vi "Noise_Tests.vi"(0 "tdms file in":refnum<k34>, 5 "Ch1_in":dbl[](array[numeric]), 7 "Ch2_in":dbl[](array[numeric]), 12 "group name":string, 13 "channel names":string[](array[string])) -> (4 "tdms file out":refnum<k34>, 6 "Ch1_out":dbl[](array[numeric]), 8 "Ch2_out":dbl[](array[numeric]), 10 "Hist":i32[][](array[numeric]), 14 "Noise Spectrum":T1(array[cluster]), 15 "Waveforms":waveform(dbl)[](array[waveform]))   [LabVIEW 2019]
uses:
  SiPM_Tests_Global_Var.vi
  <vilib>/Analysis/NI_AALPro.lvlib
  Agilent_lib/Agilent 2000 3000 X-Series.lvlib
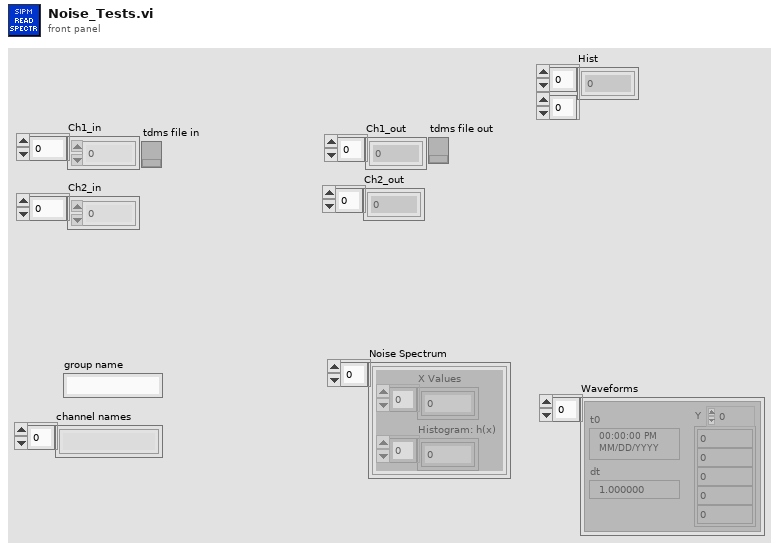
[diagram p1: front panel]
types:
  T1 = cluster{"X Values":dbl[], "Histogram: h(x)":i32[]}[]
  T2 = cluster{"X Values":dbl[], "Histogram: h(x)":i32[]}
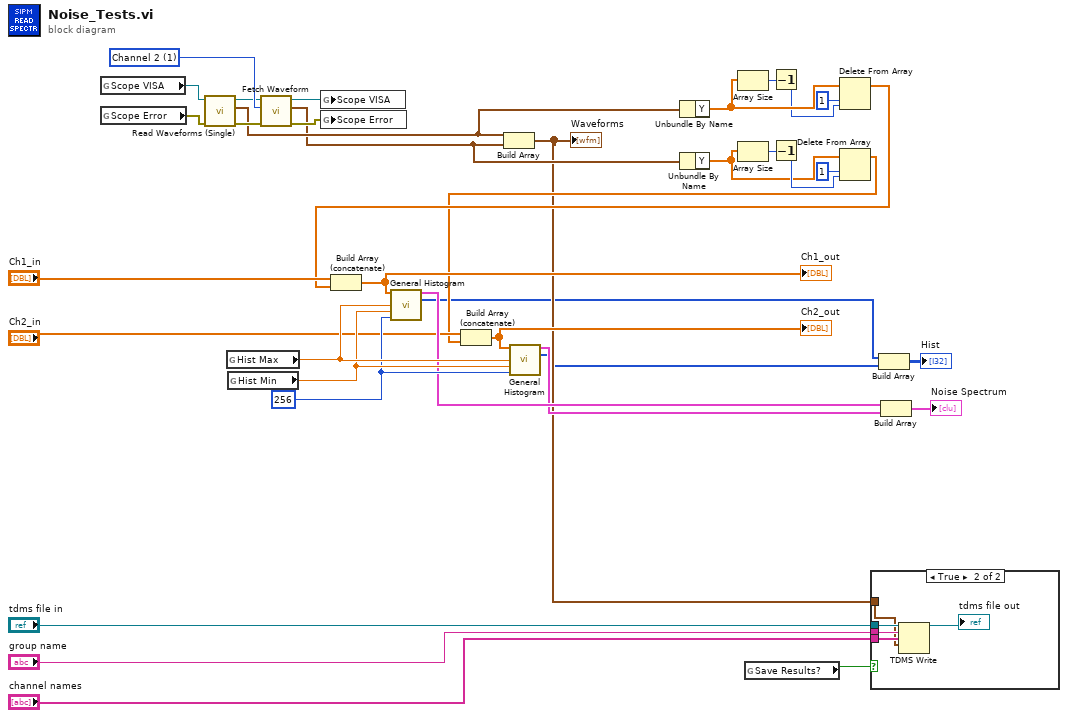
[diagram p0: block diagram]
diagram:
  w25 = 1 items=["Channel 1"=0, "Channel 2"=1, "Channel 3"=2, "Channel 4"=3, "Waveform Memory 1"=5, "Waveform Memory 2"=6, "Serial Bus 1"=7, "Serial Bus 2"=8, "Digital Bus Low"=9, "Digital Bus High "=10, "Digital Bus 1"=11, "Digital Bus 2"=12, "Function 1"=32, "Function 2"=33, "Function 3"=34, "Function 4"=35, "Math 1"=36, "Math 2"=37, "Math 3"=38, "Math 4"=39] ("Source Channel (0: Channel 1)")
  w32 = 256 ("# bins")
  n1 = global read "SiPM_Tests_Global_Var.vi" "Scope VISA"() -> (w21:refnum<visa-resource-name>)
  n2 = global read "SiPM_Tests_Global_Var.vi" "Scope Error"() -> (w22:errorcluster)
  n3 = call "Read Waveforms (Single).vi"("error in (no error)"=w22, "VISA resource name"=w21) -> ("error out"=w24:errorcluster, "Waveform Data"=w10:waveform(dbl), "VISA resource name out"=w23:refnum<visa-resource-name>)  [unwired: 7 in]
  n4 = global read "SiPM_Tests_Global_Var.vi" "Hist Max"() -> (w34:dbl)
  n5 = global read "SiPM_Tests_Global_Var.vi" "Hist Min"() -> (w33:dbl)
  n6 = call "Fetch Waveform.vi"("error in (no error)"=w24, "Source Channel (0: Channel 1)"=w25, "VISA resource name"=w23) -> ("error out"=w19:errorcluster, "Waveform Data"=w9:waveform(dbl), "VISA resource name out"=w20:refnum<visa-resource-name>)  [unwired: 2 in, 4 out]
  n7 = global write "SiPM_Tests_Global_Var.vi" "Scope VISA"(w20) -> ()
  n8 = global write "SiPM_Tests_Global_Var.vi" "Scope Error"(w19) -> ()
  n9 = Build Array(w10, w9) -> (w4:waveform(dbl)[])
  "Waveforms" <- w4
  n10 = Unbundle By Name(w10) -> ("Y"=w17:dbl[])
  n11 = Unbundle By Name(w9) -> ("Y"=w11:dbl[])
  n12 = Array Size(array=w17) -> (size(s)=w16:i32)
  n13 = Array Size(array=w11) -> (size(s)=w13:i32)
  n14 = global read "SiPM_Tests_Global_Var.vi" "Save Results?"() -> (w5:bool)
  n15 = Decrement(x=w16) -> (x-1=w15:i32)
  n16 = Decrement(x=w13) -> (x-1=w14:i32)
  n17 = Delete From Array(array=w17, length=1, index=w15) -> (array with subset deleted=w8:dbl[])  [unwired: 1 out]
  n18 = Build Array (concatenate)("Ch1_in", w8) -> (w36:dbl[])
  "Ch1_out" <- w36
  n19 = call <vilib>:"General Histogram.vi"("X"=w36, "max"=w34, "min"=w33, "# bins"=w32) -> ("Histogram Graph"=w31:T2, "Histogram"=w3:i32[])  [unwired: 7 in, 3 out]
  n20 = Delete From Array(array=w11, length=1, index=w14) -> (array with subset deleted=w6:dbl[])  [unwired: 1 out]
  n21 = Build Array (concatenate)("Ch2_in", w6) -> (w35:dbl[])
  "Ch2_out" <- w35
  n22 = call <vilib>:"General Histogram.vi"("X"=w35, "max"=w34, "min"=w33, "# bins"=w32) -> ("Histogram Graph"=w30:T2, "Histogram"=w2:i32[])  [unwired: 7 in, 3 out]
  n23 = case shown="True" w5 {
    tunnel: "tdms file in" -> [_ w41]
    tunnel: "group name" -> [_ w40]
    tunnel: "channel names" -> [_ w39]
    tunnel: w4 -> [_ w38]
    frame False {
    }
    frame True {
      n24 = TDMS Write(0:w41, 5:w40, 7:w39, 9:w38) -> (4:→"tdms file out":refnum<k34>)  [unwired: 2 in, 3 out]
    }
  }
  n25 = Build Array(w3, w2) -> (→"Hist":i32[][])
  n26 = Build Array(w31, w30) -> (→"Noise Spectrum":T1)
